vi "caget.vi"(1 "Variable":string) -> (0 "Value":string)   [LabVIEW 2010]
panel:
  out "standard error":string
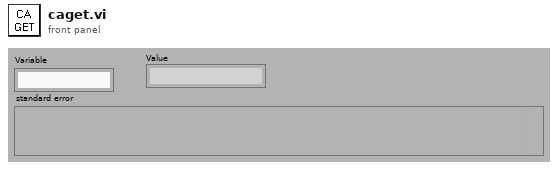
[diagram p1: front panel]
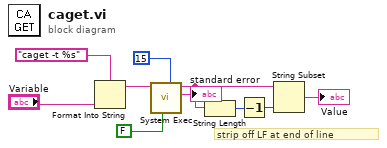
[diagram p0: block diagram]
diagram:
  # "strip off LF at end of line"
  n1 = Format Into String(format string="caget -t %s" ("Format String"), "Variable") -> (resulting string=w8:string)  [unwired: 2 in, 1 out]
  n2 = call <vilib>:"System Exec.vi"("expected output size  (4096)"=u32 15, "run minimized? (F)"=FALSE, "command line"=w8) -> ("standard error"=→"standard error":string, "standard output"=w3:string)  [unwired: 5 in, 2 out]
  n3 = String Length(string=w3) -> (length=w4:i32)
  n4 = Decrement(x=w4) -> (x-1=w5:i32)
  n5 = String Subset(string=w3, length (rest)=w5) -> (substring=→"Value":string)  [unwired: 1 in]
